vi "fgv_ublox_mainui.vi"(7 "cmd":T2, 11 "MainUI ublox":T1 {"HDOP" scale=0.0..10.0; "PDOP" scale=0.0..10.0; "2D Acc.m" scale=0.0..10.0; "Longitude" format="%.9f"; "Latitude" format="%.9f"; "3D Acc.m" scale=0.0..10.0}) -> (3 "MainUI ublox out":T1 {"HDOP" scale=0.0..10.0; "PDOP" scale=0.0..10.0; "2D Acc.m" scale=0.0..10.0; "Longitude" format="%.9f"; "Latitude" format="%.9f"; "3D Acc.m" scale=0.0..10.0})   [LabVIEW 2019]
uses:
  Ctrl/cmd_common.ctl
  Ctrl/ublox-ui_main.ctl
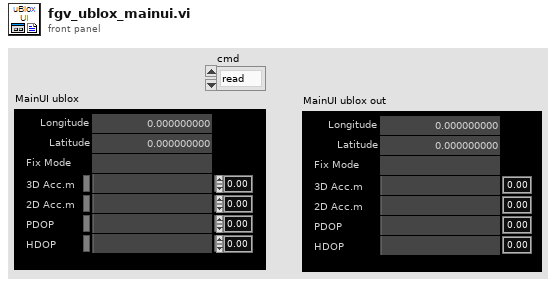
[diagram p1: front panel]
types:
  T1 = typedef "ublox-ui_main.ctl" = cluster{"Longitude  ":dbl, "Latitude     ":dbl, "Fix Mode   ":string, "3D Acc.m":dbl, "2D Acc.m":dbl, "PDOP     ":dbl, "HDOP     ":dbl}
  T2 = typedef "cmd_common.ctl" = enum16{"read", "write"}
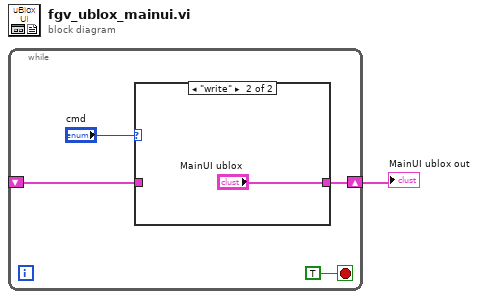
[diagram p0: block diagram]
diagram:
  n1 = while {
    shift-right: [w3] -> w1
    shift-left: _ -> [w2]
    stop <- TRUE stop-if-true
    n2 = case shown="\"write\"" "cmd" {
      tunnel: [w6 "MainUI ublox"] -> w3
      tunnel: w2 -> [w6 _]
      frame "read", Default {
      }
      frame "write" {
      }
    }
  }
  "MainUI ublox out" <- w1
